vi "Write Event From Sink Abstract Msg Msg.vi"(10 "Event Source.lvlib:Event From Sink Abstract Msg Msg.lvclass":refnum<class "Event From Sink Abstract Msg Msg.lvclass">=refnum, 11 "Event Source in":refnum<class "Event Source.lvclass">) -> (3 "Event Source out":refnum<class "Event Source.lvclass">)   [LabVIEW 2016]
uses:
  Event Source.lvclass
  C:/Program Files (x86)/National Instruments/LabVIEW 2016/vi.lib/ActorFramework/Actor/Actor.lvclass
  Event Source Messages/Event From Sink Abstract Msg Msg/Event From Sink Abstract Msg Msg.lvclass
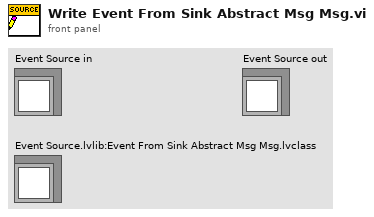
[diagram p1: front panel]
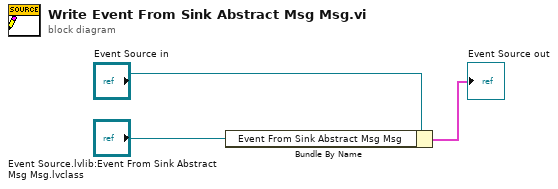
[diagram p0: block diagram]
diagram:
  n1 = Bundle By Name(cluster="Event Source in", "Event From Sink Abstract Msg Msg"="Event Source.lvlib:Event From Sink Abstract Msg Msg.lvclass") -> (→"Event Source out":cluster{})
